vi "Read.vi"(8 "error in (no error)":errorcluster caption="entrée d'erreur (pas d'erreur)", 11 "Class UART (Default) en entrée":refnum<class "Class UART P2056.lvclass">) -> (0 "error out":errorcluster caption="sortie d'erreur", 3 "Class UART (Default) en sortie":refnum<class "Class UART P2056.lvclass">)   [LabVIEW 2020, in "Library Instrument & Equipement.lvlib" / "Library UART.lvlib" / "Class UART P2056.lvclass"]
uses:
  Class UART P2056.lvclass
  C:/Users/ngarcin/OneDrive - Altyor/Standard TB/Class/UART/UART (Default)/Class UART (Default).lvclass
  Class UART P2056.lvclass/Class UART P2056.ctl
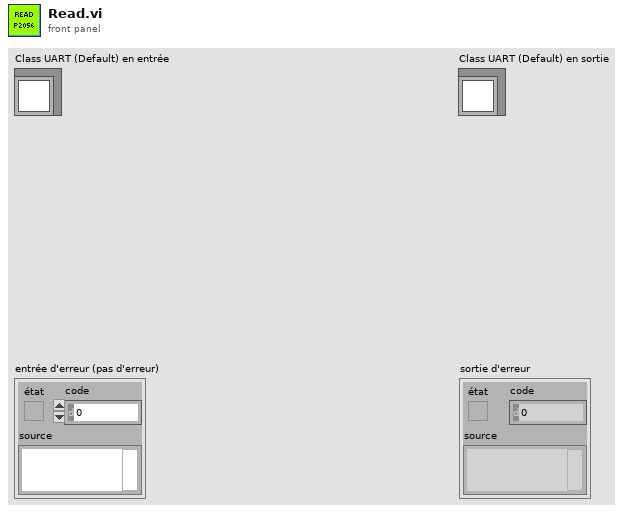
[diagram p1: front panel]
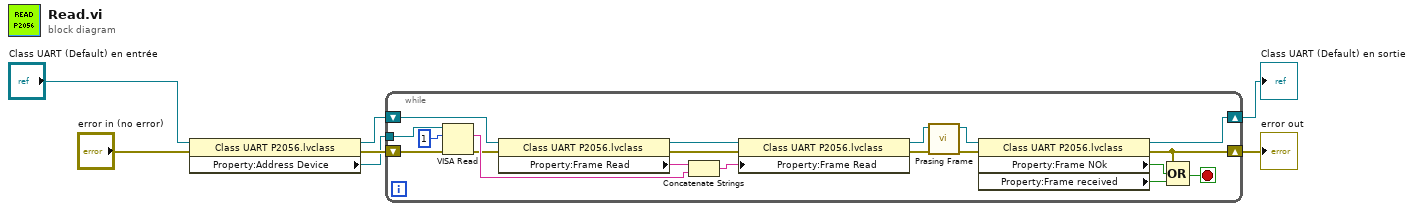
[diagram p0: block diagram]
diagram:
  n1 = property class="Class UART P2056.lvclass"(reference="Class UART (Default) en entrée", error in="error in (no error)") -> (reference out=w2:refnum<class "Class UART P2056.lvclass">, error out=w4:errorcluster, "Property:Address Device"=w3:refnum<visa-resource-name>)
  n2 = while {
    tunnel: w3 -> [w21]
    shift-right: [w8] -> w7
    shift-left: w4 -> [w22]
    shift-right: [w9] -> w6
    shift-left: w2 -> [w19]
    stop <- w20 stop-if-true
    n3 = VISA Read(VISA resource name=w21, byte count=u32 1 ("nombre d'octets"), error in (no error)=w22) -> (read buffer=w14:string, error out=w10:errorcluster)  [unwired: 2 out]
    n4 = property class="Class UART P2056.lvclass"(reference=w19, error in=w10) -> (reference out=w17:refnum<class "Class UART P2056.lvclass">, error out=w16:errorcluster, "Property:Frame Read"=w15:string)
    n5 = Concatenate Strings(w15, w14) -> (w13:string)
    n6 = property class="Class UART P2056.lvclass"(reference=w17, error in=w16, "Property:Frame Read"=w13) -> (reference out=w11:refnum<class "Class UART P2056.lvclass">, error out=w12:errorcluster)
    n7 = call-dynamic "Prasing Frame.vi"("error in (no error)"=w12, "Class UART Enocean en entrée"=w11) -> ("error out"=w25:errorcluster, "Class UART Enocean en sortie"=w26:refnum<class "Class UART P2056.lvclass">)  [unwired: 8 in]
    n8 = property class="Class UART P2056.lvclass"(reference=w26, error in=w25) -> (reference out=w9:refnum<class "Class UART P2056.lvclass">, error out=w8:errorcluster, "Property:Frame NOk"=w24:bool, "Property:Frame received"=w23:bool)
    n9 = Compound Arithmetic op=OR ("Opérateur arithmétique")(w8, w24, w23) -> (w20:bool)
  }
  "error out" <- w7
  "Class UART (Default) en sortie" <- w6
